vi "Constants.vi"() -> ()   [LabVIEW 2017, in "Data Sharing Custom Device Shared.lvlib"]
doc: "Use this Global VI to access the GUIDs assigned to the page resources of the Custom Device."
uses:
  Data Sharing Custom Device Shared.lvlib
panel:
  in  "Tab Control":enum32{"GUIDS", "Constants", "Properties"}(tab)
  in  "Extra 2":string="58daca15-92db-4c93-a3ad-b73ea18fd830"
  in  "Extra 1":string="fac80506-817b-428b-b621-f92416c1df4e"
  in  "Extra 0":string="aa8f3574-ac18-44db-994c-aaee51b3c8c2"
  in  "Settings":string="5cb8cfdf-a02f-4ef9-851e-4d7766c2100a"
  in  "Channel":string="e2292671-c630-4eec-8542-8794c1c5e9f3"
  in  "Transfer":string="da89d37c-3698-4b07-8aa7-3d84bcbf2809"
  in  "Transfer Group":string="c4ceb080-9927-4f6e-8024-6d8bd670f2a9"
  in  "Plugin":string="21d3fd0c-cd96-460d-bfd7-1220a208cdb3"
  in  "Framework":string="9ea28b24-382c-4156-8b1a-a9fa1bfd7c2d"
  in  "Data Sharing Custom Device":string="5a136c0f-7458-47a6-ba75-b1abd87bd209"
  in  "Compiled.Settings":string="Compiled.Settings"
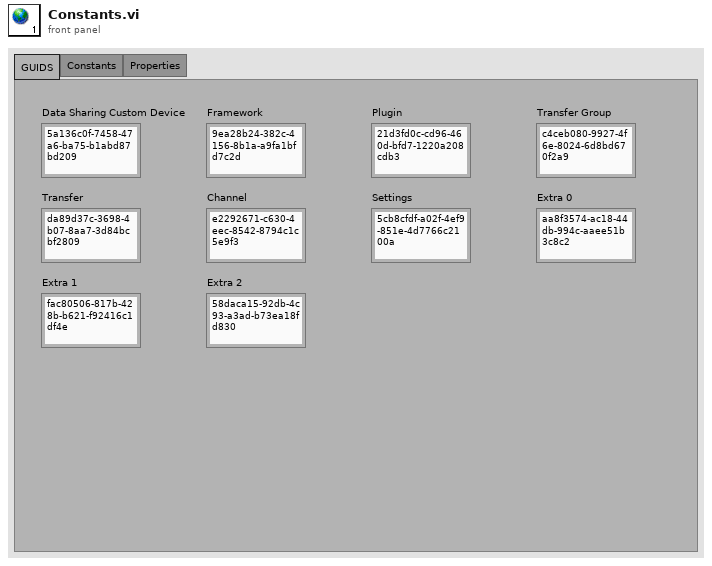
[diagram p1: front panel]
diagram:
